vi "Untitled 2 (SubVI).vi"(11 "mean":dbl) -> (3 "T":dbl)   [LabVIEW 2023]
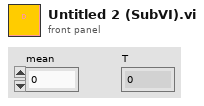
[diagram p1: front panel]
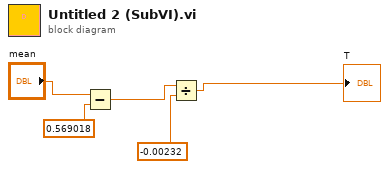
[diagram p0: block diagram]
diagram:
  n1 = Subtract(x="mean", y=0.569018) -> (x-y=w3:dbl)
  n2 = Divide(x=w3, y=-0.00232) -> (x/y=→"T":dbl)
